vi "DUAL GAUGE-ConverIntIntEngEng.vi"(0 "String in":string) -> (6 "Integer1 out":u8, 8 "Eng1 out":dbl format="%.3e", 10 "Integer2 out":u8, 15 "Eng2 out":dbl format="%.3e")   [LabVIEW 2010, in "Dual Gauge.lvlib"]
uses:
  Dual Gauge.lvlib
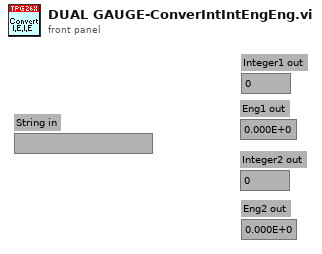
[diagram p1: front panel]
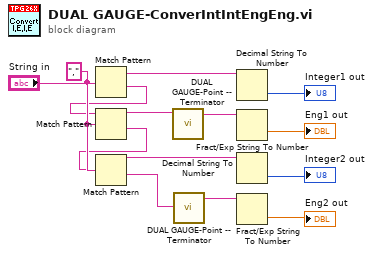
[diagram p0: block diagram]
diagram:
  w10 = "," ("regular expression")
  n1 = Match Pattern(string="String in", regular expression=w10) -> (before substring=w5:string, after substring=w6:string)  [unwired: 1 in, 2 out]
  n2 = Match Pattern(string=w6, regular expression=w10) -> (before substring=w11:string, after substring=w9:string)  [unwired: 1 in, 2 out]
  n3 = Match Pattern(string=w9, regular expression=w10) -> (before substring=w3:string, after substring=w2:string)  [unwired: 1 in, 2 out]
  n4 = call "DUAL GAUGE-Point -- Terminator.vi"("Eingangstring"=w11) -> ("Ausgangstring"=w8:string)
  n5 = call "DUAL GAUGE-Point -- Terminator.vi"("Eingangstring"=w2) -> ("Ausgangstring"=w7:string)
  n6 = Decimal String To Number(string=w5) -> (number=→"Integer1 out":i32)  [unwired: 2 in, 1 out]
  n7 = Fract/Exp String To Number(string=w8) -> (number=→"Eng1 out":dbl)  [unwired: 3 in, 1 out]
  n8 = Decimal String To Number(string=w3) -> (number=→"Integer2 out":i32)  [unwired: 2 in, 1 out]
  n9 = Fract/Exp String To Number(string=w7) -> (number=→"Eng2 out":dbl)  [unwired: 3 in, 1 out]
